vi "Read Configuration-json.vi"(8 "error in (no error)":errorcluster, 11 "Filename":string="myDAQConfi.ini") -> (0 "error out":errorcluster, 1 "isDeviceExist":bool, 3 "Configuration":T5)   [LabVIEW 2016]
uses:
  Control/Configuration.ctl
  Control/TaskConfig.ctl
  Control/ChanConfig.ctl
  Control/ClockConfig.ctl
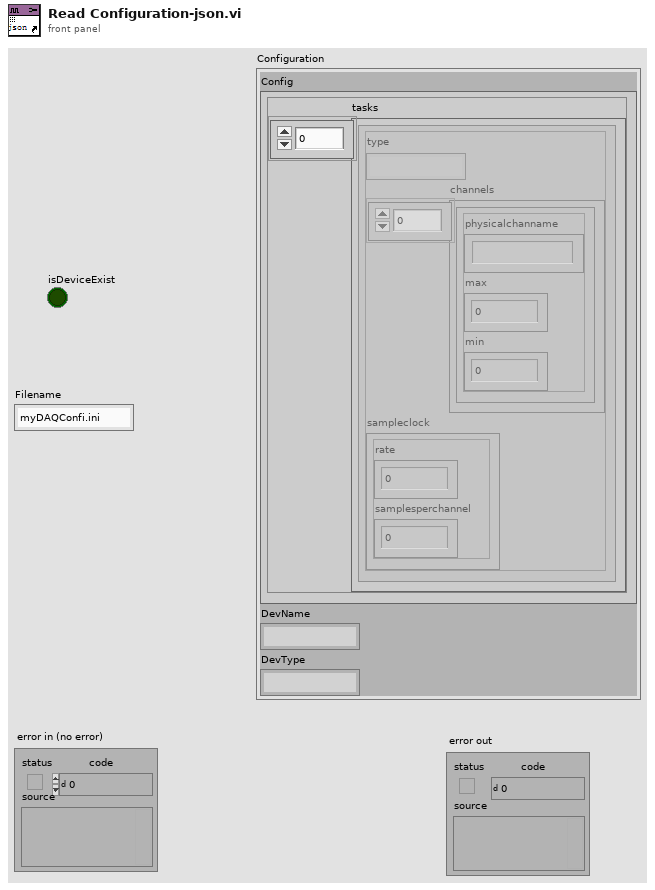
[diagram p1: front panel]
types:
  T1 = typedef "Configuration.ctl" = cluster{"tasks":T2[]}
  T2 = typedef "TaskConfig.ctl" = cluster{"type":string, "channels":T3[], "sampleclock":T4}
  T3 = typedef "ChanConfig.ctl" = cluster{"physicalchanname":string, "max":dbl, "min":dbl}
  T4 = typedef "ClockConfig.ctl" = cluster{"rate":dbl, "samplesperchannel":i32}
  T5 = cluster{"Config":T1, "DevName":string, "DevType":string}
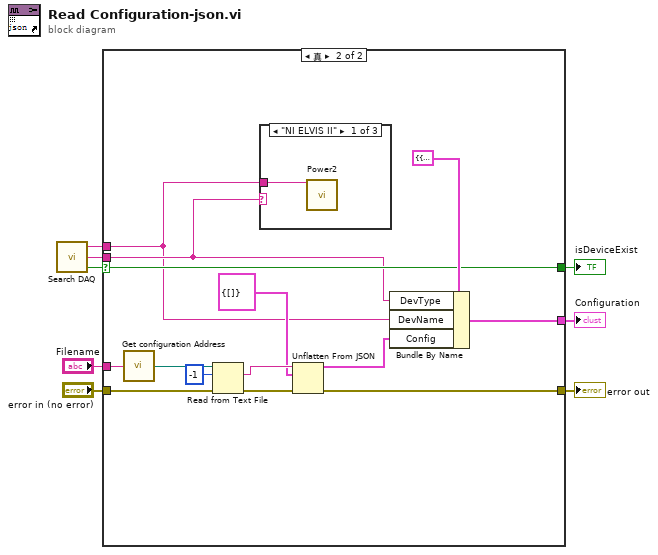
[diagram p0: block diagram]
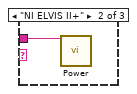
[diagram p3: hidden frame]
diagram:
  n1 = call "Search DAQ.vi"() -> ("Dev"=w1:tag, "ProductType"=w2:string, "isDevExist？"=w5:bool)  [unwired: 7 in]
  n2 = case shown="真" w5 {
    selector: w5 -> [w9 w16]
    tunnel: "Filename" -> [_ w24]
    tunnel: "error in (no error)" -> [w10 w22]
    tunnel: [w10 w19] -> w6
    tunnel: w1 -> [_ w12]
    tunnel: [_ w17] -> w3
    tunnel: [w9 w16] -> w4
    tunnel: w2 -> [_ w13]
    frame False {
    }
    frame True {
      n3 = call "Get configuration Address.vi"("文件名"=w24) -> ("配置文件路径"=w11:path)
      n4 = Read from Text File(file (use dialog)=w11, count=-1 ("计数"), error in=w22) -> (text=w21:string, error out=w20:errorcluster)  [unwired: 1 in, 2 out]
      n5 = case shown="\"NI ELVIS II\"" w13 {
        tunnel: w12 -> [w25 w26 _]
        frame "NI ELVIS II" {
          n6 = call "Power2"("Device Name"=w25) -> ()  [unwired: 16 in, 3 out]
        }
        frame "NI ELVIS II+" {
          n7 = call "Power"("Device Name"=w26) -> ()  [unwired: 16 in, 3 out]
        }
        frame "NI myDAQ", Default {
        }
      }
      n8 = Unflatten From JSON(JSON string=w21, type and defaults=T1 {"tasks"=[]} ("Configuration"), error in (no error)=w20) -> (value=w15:T1, error out=w19:errorcluster)  [unwired: 4 in]
      n9 = Bundle By Name(cluster=T5 {"Config"={"tasks"=[]}, "DevName"="", "DevType"=""}, "DevType"=w13, "DevName"=w12, "Config"=w15) -> (w17:T5)
    }
  }
  "error out" <- w6
  "isDeviceExist" <- w4
  "Configuration" <- w3
